vi "Lua palette file path.vi"() -> (3 "palette file path":path)   [LabVIEW 2020, in "Lua DevUtil.lvlib"]
uses:
  Lua DevUtil.lvlib
  Lua for LabVIEW/Lua/New Lua State.vi
  Lua for LabVIEW/Lua/Lua.lvclass
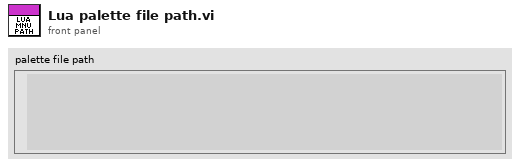
[diagram p1: front panel]
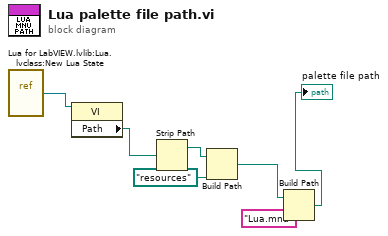
[diagram p0: block diagram]
diagram:
  n1 = vi-ref "Lua for LabVIEW.lvlib:Lua.lvclass:New Lua State.vi"() -> (w7:refnum<vi>)
  n2 = property class="VI"(reference=w7) -> ("Path"=w6:path)  [unwired: 1 in, 2 out]
  n3 = Strip Path(path=w6) -> (stripped path=w5:path)  [unwired: 1 out]
  n4 = Build Path(base path=w5, name or relative path=path "resources") -> (appended path=w3:path)
  n5 = Build Path(base path=w3, name or relative path="Lua.mnu") -> (appended path=→"palette file path":path)
